vi "Initialize Array Activity.vi"() -> ()   [LabVIEW 2014]
panel:
  out "?":dbl[][](array[numeric])
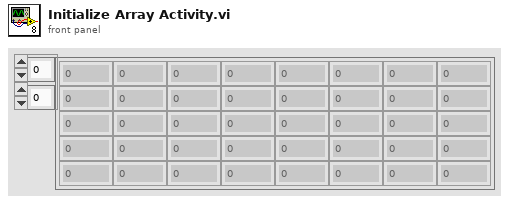
[diagram p1: front panel]
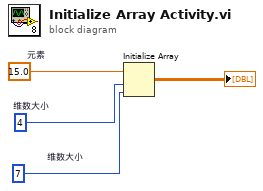
[diagram p0: block diagram]
diagram:
  w2 = 7  # 维数大小
  w3 = 4  # 维数大小
  w4 = 15.0  # 元素
  n1 = Initialize Array(w4, w3, w2) -> (→"?":dbl[][])
